vi "Write CtrlType.vi"(8 "error in (no error)":errorcluster, 10 "IO Card Type":T1, 11 "AxisCard in":refnum<class "AxisCard.lvclass">) -> (0 "error out":errorcluster, 3 "AxisCard out":refnum<class "AxisCard.lvclass">)   [LabVIEW 2019, in "AxisCard.lvclass"]
uses:
  AxisCard.lvclass
  IO Folder/IO_VI/IOCtrl/Ctrl/IO Card_Type.ctl
  AxisCard.lvclass/AxisCard.ctl
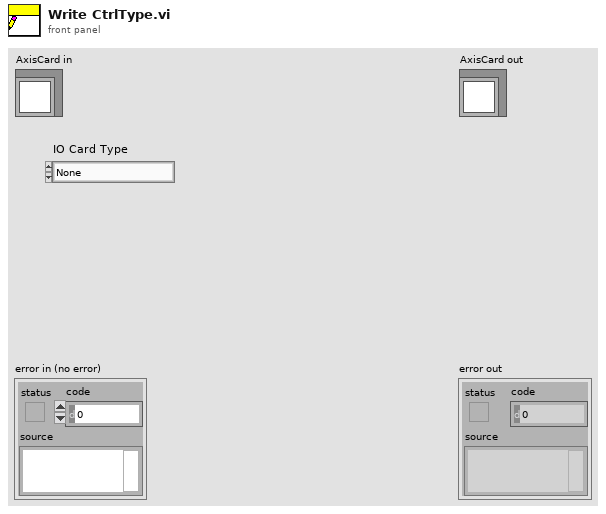
[diagram p1: front panel]
types:
  T1 = typedef "IO Card_Type.ctl" = enum16{"None", "Unidaq32", "6480", "2410C-64", "Zan", "DMC1000B", "16InOut", "Robot", "DMC3600"}
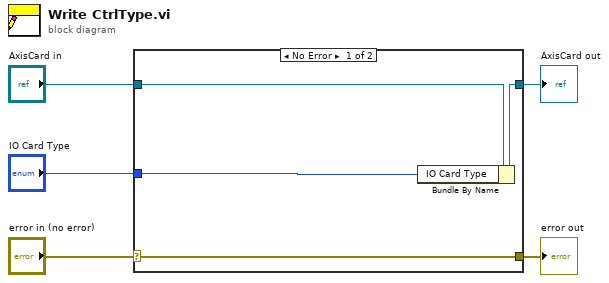
[diagram p0: block diagram]
diagram:
  n1 = case shown="No Error" "error in (no error)" {
    selector: "error in (no error)" -> [w9 w10]
    tunnel: [w9 w10] -> w4
    tunnel: [w7 w11] -> w2
    tunnel: "AxisCard in" -> [w8 w11]
    tunnel: "IO Card Type" -> [w6 _]
    frame No Error {
      n2 = Bundle By Name(cluster=w8, "IO Card Type"=w6) -> (w7:refnum<class "AxisCard.lvclass">)
    }
    frame Error {
    }
  }
  "error out" <- w4
  "AxisCard out" <- w2
